vi "通用报警缓存文件名.vi"(7 "报警类型":enum16{"剂量率报警", "累积剂量报警"}(ring), 10 "时值":T1, 11 "名称":string) -> (3 "文件名":string caption="结果")   [LabVIEW 2017]
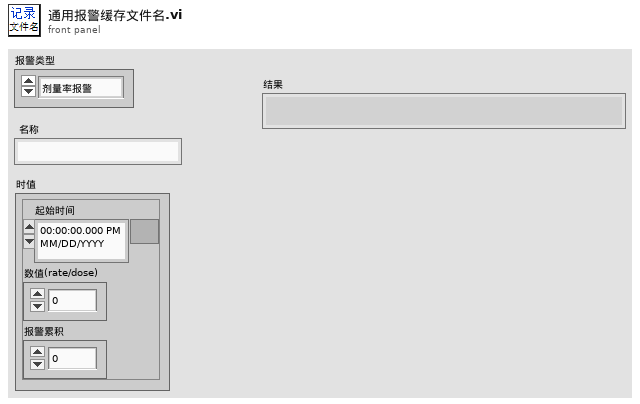
[diagram p1: front panel]
types:
  T1 = cluster{"起始时间":timestamp, "数值(rate/dose)":dbl, "报警累积":dbl}
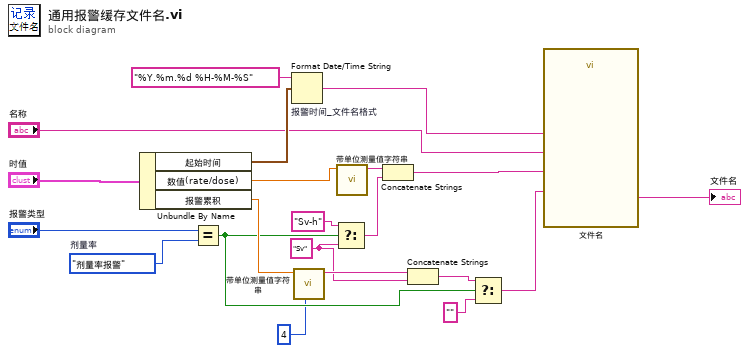
[diagram p0: block diagram]
diagram:
  w6 = "Sv" ("字符串")
  w18 = enum16{"剂量率报警", "累积剂量报警"}."剂量率报警"  # 剂量率
  n1 = Unbundle By Name("时值") -> ("起始时间"=w14:timestamp, "数值(rate/dose)"=w13:dbl, "报警累积"=w8:dbl)
  n2 = Equal?(x="报警类型", y=w18) -> (x = y?=w5:bool)
  n3 = Format Date/Time String "报警时间_文件名格式"(time format string (%c)="%Y.%m.%d %H-%M-%S" ("时间格式字符串(%c)"), seconds (now)=w14) -> (date/time string=w12:string)  [unwired: 1 in]
  n4 = call "带单位测量值字符串.vi"("精度(2)"=i16 4, "测量值"=w8) -> ("结果"=w7:string)  [unwired: 9 in]
  n5 = Select(t="Sv-h" ("字符串"), s=w5, f=w6) -> (s? t:f=w16:string)
  n6 = call "带单位测量值字符串.vi"("测量值"=w13) -> ("结果"=w20:string)  [unwired: 10 in]
  n7 = Concatenate Strings(w20, w16) -> (w10:string)
  n8 = Concatenate Strings(w7, w6) -> (w4:string)
  n9 = Select(t=w4, s=w5, f="") -> (s? t:f=w2:string)
  n10 = call "文件名"("报警累积"=w2, "日期"=w12, "名称"="名称", "报警值"=w10) -> ("Result"=→"文件名":string)  [unwired: 10 in, 1 out]
